vi "wait for recovered modules.vi"(5 "worker pool reference":T2, 7 "fault fifo":refnum<k33>, 8 "error in":errorcluster, 9 "time data in":T1, 10 "run flags in":u8[](array[numeric]), 11 "modules in":T5[](array[typedef]) {"GUID"."Lo" format="%.0x"; "GUID"."Hi" format="%.0x"}) -> (0 "error out":errorcluster, 2 "run flags out":u8[](array[numeric]), 3 "modules out":T5[](array[typedef]) {"GUID"."Lo" format="%.0x"; "GUID"."Hi" format="%.0x"})   [LabVIEW 2013, in "main engine.lvlib"]
uses:
  main engine/main engine.lvlib
  full module data.ctl
  <vilib>/NI/Tag Bus Module Framework/runtime/TBM module execution interface.lvclass
  module run state.ctl
  async executor/asynchronous executor reference.ctl
  async executor/message to executor.ctl
  async command notification.ctl
  <vilib>/NI/Tag Bus/table/data table.ctl
  async error info.ctl
  <vilib>/NI/Tag Bus Module Framework/runtime/error classification.ctl
  <vilib>/NI/Tag Bus/buffer exchange/buffer reference.ctl
  <vilib>/NI/Tag Bus Module Framework/module configuration/TBM module configuration.lvclass
  <vilib>/NI/Configuration Framework/serializable configuration/Numeric GUID.ctl
  module method data.ctl
  <vilib>/NI/Tag Bus/table/transfer specification.ctl
  <vilib>/NI/Tag Bus/tag/Data Type.ctl
  fault handling spec.ctl
  Configuration/Error Actions.ctl
  worker library/worker comms.ctl
  worker library/worker commands.ctl
  worker library/request fifos.ctl
  worker library/recovery request.ctl
  worker library/response fifos.ctl
  worker library/recovery response.ctl
  rt fault.ctl
  time information.ctl
  worker library/worker pool.lvlib
  <vilib>/NI/Tag Bus/table/data table.lvlib
  <vilib>/NI/Tag Bus/buffer exchange/tag bus buffer exchange.lvlib
  async executor/async executor.lvlib
  <vilib>/NI/Tag Bus/tag/tag descriptor.lvclass
  Configuration/Standard Engine Configuration.lvclass
  <vilib>/NI/Configuration Framework/serializable configuration/NISE_CEF_serializable configuration.lvclass
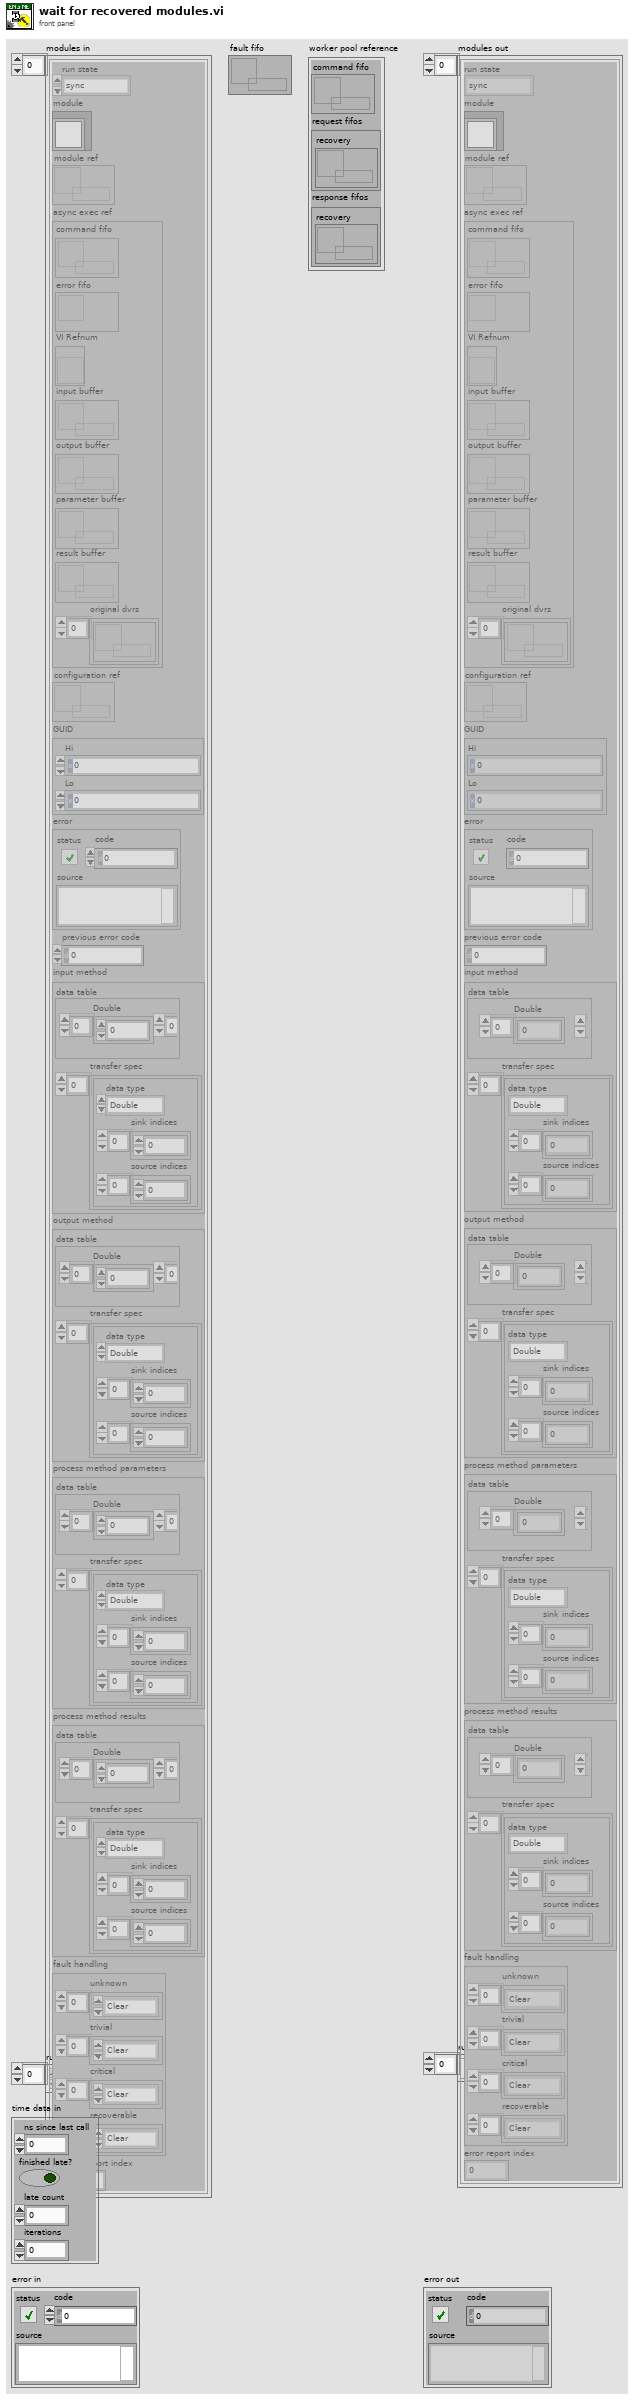
[diagram p1: front panel]
types:
  T1 = typedef "main engine.lvlib/time information.ctl" = cluster{"ns since last call":u64, "finished late?":bool, "late count":u32, "iterations":u64}
  T2 = typedef "worker pool.lvlib/worker comms.ctl" = cluster{"command fifo":refnum<k33>, "request fifos":T3, "response fifos":T4}
  T3 = typedef "worker pool.lvlib/request fifos.ctl" = cluster{"recovery":refnum<k33>}
  T4 = typedef "worker pool.lvlib/response fifos.ctl" = cluster{"recovery":refnum<k33>}
  T5 = typedef "main engine.lvlib/full module data.ctl" = cluster{"run state":T6, "module":refnum<class "TBM module execution interface.lvclass">, "module ref":refnum<data-value>, "async exec ref":T7, "configuration ref":refnum<data-value>, "GUID":T9, "error":errorcluster, "previous error code":i32, "input method":T10, "output method":T10, "process method parameters":T10, "process method results":T10, "fault handling":T14, "error report index ":i32}
  T6 = typedef "main engine.lvlib/module run state.ctl" = enum16{"sync", "async"}
  T7 = typedef "async executor.lvlib/asynchronous executor reference.ctl" = cluster{"command fifo":refnum<k33>, "error fifo":refnum<k33>, "VI Refnum":refnum<vi>, "input buffer":refnum<k33>, "output buffer":refnum<k33>, "parameter buffer":refnum<k33>, "result buffer":refnum<k33>, "original dvrs":T8[]}
  T8 = typedef "tag bus buffer exchange.lvlib/buffer reference.ctl" = refnum<data-value>
  T9 = typedef "NISE_CEF_serializable configuration.lvclass/Numeric GUID.ctl" = cluster{"Hi":u64, "Lo":u64}
  T10 = typedef "main engine.lvlib/module method data.ctl" = cluster{"data table":T11, "transfer spec":T12[]}
  T11 = typedef "tag bus.lvlib/data table.lvlib/data table.ctl" = cluster{"Double":dbl[], "Single":sgl[], "I64":i64[], "I32":i32[], "I16":i16[], "I8":i8[], "U64":u64[], "U32":u32[], "U16":u16[], "U8":u8[], "Boolean":bool[], "String":string[], "Array of Double":cluster{"DBL Array":dbl[]}[], "Array of Single":cluster{"SGL Array":sgl[]}[], "Array of I64":cluster{"I64 Array":i64[]}[], "Array of I32":cluster{"I32 Array":i32[]}[], "Array of I16":cluster{"I16 Array":i16[]}[], "Array of I8":cluster{"I8 Array":i8[]}[], "Array of U64":cluster{"U64 Array":u64[]}[], "Array of U32":cluster{"U32 Array":u32[]}[], "Array of U16":cluster{"U16 Array":u16[]}[], "Array of U8":cluster{"U8 Array":u8[]}[], "Array of Boolean":cluster{"Boolean Array":bool[]}[], "Array of String":cluster{"String Array":string[]}[]}
  T12 = typedef "tag bus.lvlib/data table.lvlib/transfer specification.ctl" = cluster{"data type":T13, "sink indices":i32[], "source indices":i32[]}
  T13 = typedef "tag bus.lvlib/tag descriptor.lvclass/Data Type.ctl" = enum16{"Double", "Single", "I64", "I32", "I16", "I8", "U64", "U32", "U16", "U8", "Boolean", "String", "Array of Double", "Array of Single", "Array of I64", "Array of I32", "Array of I16", "Array of I8", "Array of U64", "Array of U32", "Array of U16", "Array of U8", "Array of Boolean", "Array of String"}
  T14 = typedef "main engine.lvlib/fault handling spec.ctl" = cluster{"unknown":T15[], "trivial":T15[], "critical":T15[], "recoverable":T15[]}
  T15 = typedef "Standard Engine Configuration.lvclass/Error Actions.ctl" = enum16{"Clear", "Notify", "Stop Component", "Stop Engine", "Safe State", "Attempt Recovery"}
  T16 = typedef "worker pool.lvlib/recovery response.ctl" = cluster{"module ref":refnum<data-value>, "engine reference":i32, "original run flags":u8, "success?":bool, "error code":i32}
  T17 = typedef "TBM module execution interface.lvclass/error classification.ctl" = enum16{"unknown", "none", "trivial", "recoverable", "critical"}
  T18 = typedef "main engine.lvlib/rt fault.ctl" = cluster{"code":i32, "classification":T17, "iteration":u64, "cfg ref":refnum<data-value>}
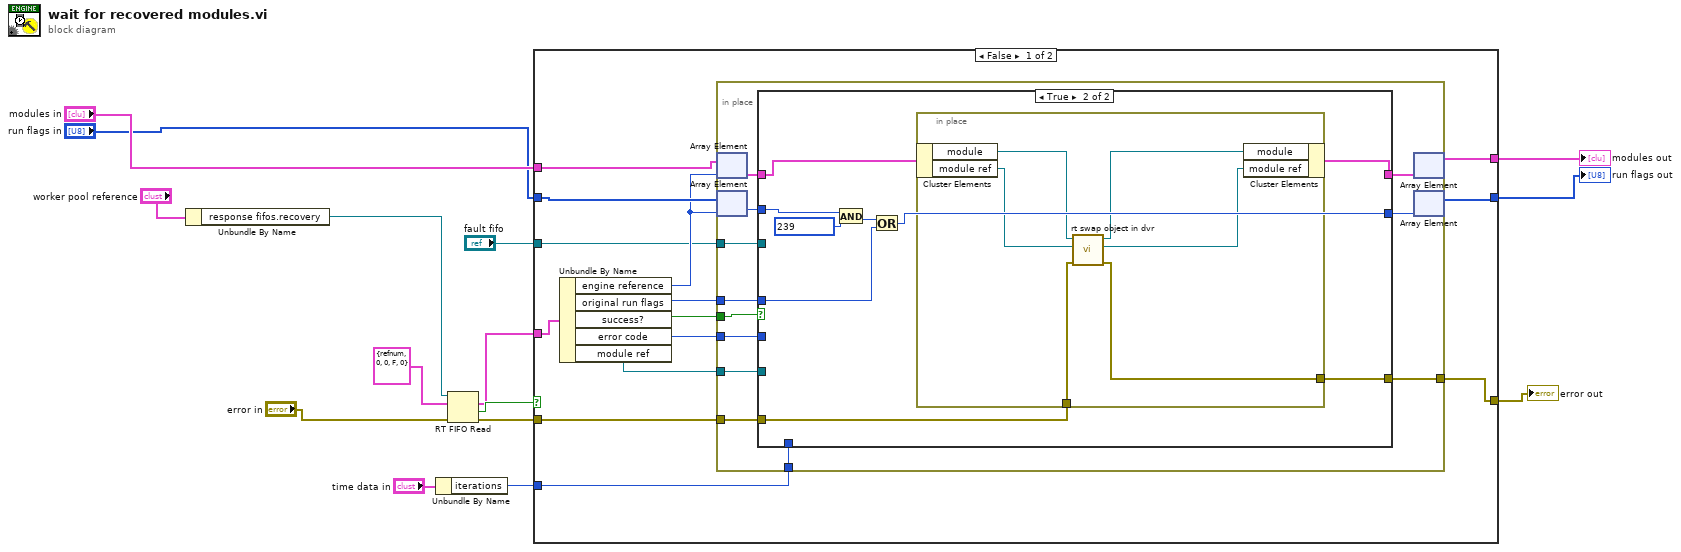
[diagram p0: block diagram]
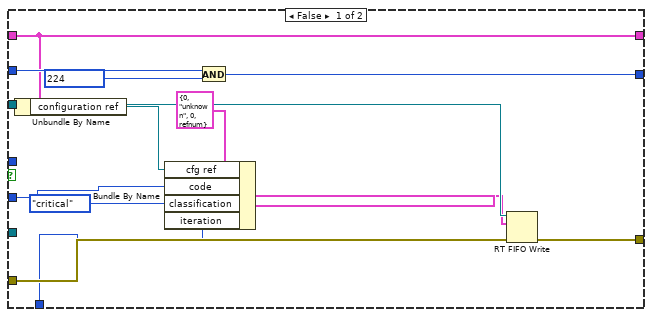
[diagram p2: hidden frame]
diagram:
  n1 = Unbundle By Name("worker pool reference") -> ("response fifos.recovery"=w13:refnum<k33>)
  n2 = Unbundle By Name("time data in") -> ("iterations"=w2:u64)
  n3 = RT FIFO Read(0:w13, 1:T16 {"module ref"=refnum, "engine reference"=0, "original run flags"=0, "success?"=FALSE, "error code"=0} ("element"), 3:"error in") -> (9:w5:T16, 10:w12:bool, 11:w10:errorcluster)  [unwired: 1 in, 2 out]
  n4 = case shown="False" w12 {
    tunnel: [w21 w72] -> w11
    tunnel: w10 -> [w20 w72]
    tunnel: "modules in" -> [w28 w71]
    tunnel: [w25 w71] -> w8
    tunnel: [w26 w70] -> w7
    tunnel: "run flags in" -> [w27 w70]
    tunnel: w5 -> [w29 _]
    tunnel: "fault fifo" -> [w19 _]
    tunnel: w2 -> [w17 _]
    frame False {
      n5 = Unbundle By Name(w29) -> ("engine reference"=w24:i32, "original run flags"=w22:u8, "success?"=w23:bool, "error code"=w18:i32, "module ref"=w16:refnum<data-value>)
      n6 = in-place {
        in-place-border: w23 -> [w41]
        in-place-border: w22 -> [w34]
        in-place-border: [w36] -> w21
        in-place-border: w20 -> [w35]
        in-place-border: w19 -> [w33]
        in-place-border: w18 -> [w32]
        in-place-border: w17 -> [w31]
        in-place-border: w16 -> [w30]
        n7 = in-place-array #1(w28, w24) -> (w39:T5)
        n8 = in-place-array #2(w27, w24) -> (w38:u8)
        n9 = case shown="True" w41 {
          tunnel: [w42 w57] -> w40
          tunnel: w39 -> [w42 w58]
          tunnel: w38 -> [w54 w63]
          tunnel: [w52 w59] -> w37
          tunnel: [w50 w55] -> w36
          tunnel: w35 -> [w51 w56]
          tunnel: w34 -> [_ w60]
          tunnel: w33 -> [w49 _]
          tunnel: w32 -> [w46 _]
          tunnel: w31 -> [w45 _]
          tunnel: w30 -> [_ _]
          frame False {
            n10 = Unbundle By Name(w42) -> ("configuration ref"=w43:refnum<data-value>)
            n11 = Bundle By Name(cluster=T18 {"code"=0, "classification"=enum."unknown", "iteration"=0, "cfg ref"=refnum} ("element"), "cfg ref"=w43, "code"=w46, "classification"=error_classification."critical", "iteration"=w45) -> (w47:T18)
            n12 = And(x=w54, y=u8 224) -> (x .and. y?=w52:u8)
            n13 = RT FIFO Write(0:w49, 1:w47, 3:w51) -> (11:w50:errorcluster)  [unwired: 2 in, 3 out]
          }
          frame True {
            n14 = And(x=w63, y=u8 239) -> (x .and. y?=w61:u8)
            n15 = Or(x=w61, y=w60) -> (x .or. y?=w59:u8)
            n16 = in-place {
              in-place-border: w56 -> [w65]
              in-place-border: [w64] -> w55
              n17 = in-place-cluster #3(w58) -> ("module"=w69:refnum<class "TBM module execution interface.lvclass">, "module ref"=w66:refnum<data-value>)
              n18 = call "rt swap object in dvr.vi"("error in"=w65, "module ref in in"=w66, "module in"=w69) -> ("error out"=w64:errorcluster, "module ref out"=w67:refnum<data-value>, "module out"=w68:refnum<class "TBM module execution interface.lvclass">)  [unwired: 6 in]
              n19 = in-place-cluster #3("module"=w68, "module ref"=w67) -> (w57:T5)
            }
          }
        }
        n20 = in-place-array #1(w40) -> (w25:T5[])  [unwired: 1 out]
        n21 = in-place-array #2(w37) -> (w26:u8[])  [unwired: 1 out]
      }
    }
    frame True {
    }
  }
  "error out" <- w11
  "run flags out" <- w7
  "modules out" <- w8
